vi "atMonochromator_getEvent_SettingsAppliedMonochromatorRanges.vi"(8 "error in (no error)":errorcluster, 11 "logevent_SettingsAppliedMonochromatorRanges_Ctl":T1) -> (0 "error out":errorcluster, 2 "function return":i32, 3 "logevent_SettingsAppliedMonochromatorRanges_Ctl out":T1)   [LabVIEW 2016, in "SALLV_atMonochromator.lvlib"]
doc: "int atMonochromator_shm_getEvent_SettingsAppliedMonochromatorRangesLV(atMonochromator_logevent_SettingsAppliedMonochromatorRangesLV *logevent_SettingsAppliedMonochromatorRanges_Ctl );"
uses:
  SALLV_atMonochromator.lvlib
  DataTypes/logevent_SettingsAppliedMonochromatorRanges.ctl
  SALLV_atMonochromator.so
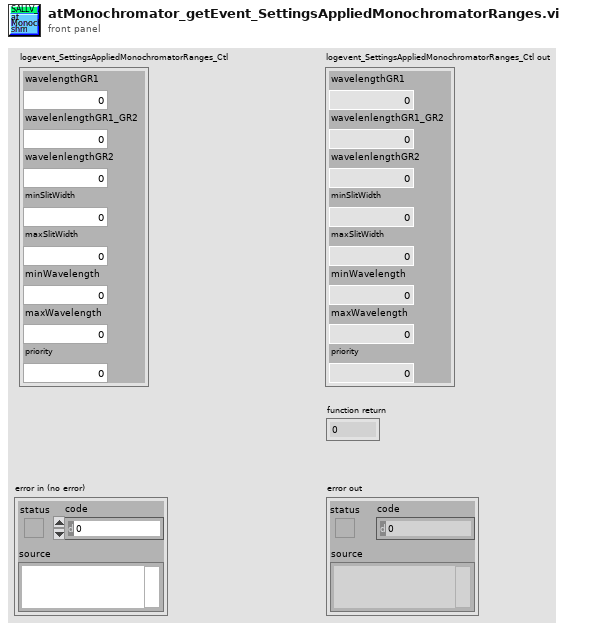
[diagram p1: front panel]
types:
  T1 = typedef "SALLV_atMonochromator.lvlib/logevent_SettingsAppliedMonochromatorRanges.ctl" = cluster{"wavelengthGR1":sgl, "wavelenlengthGR1_GR2":sgl, "wavelenlengthGR2":sgl, "minSlitWidth":sgl, "maxSlitWidth":sgl, "minWavelength":sgl, "maxWavelength":sgl, "priority":i32}
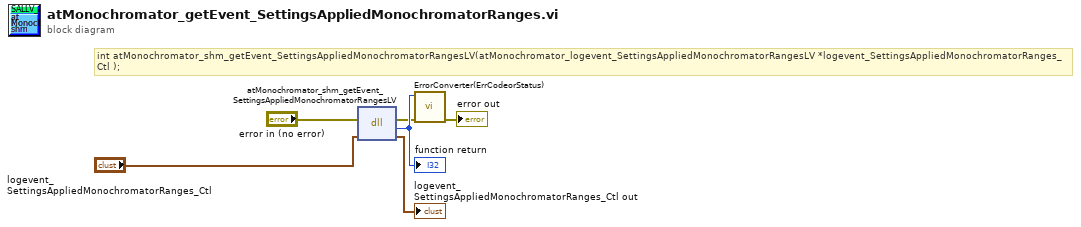
[diagram p0: block diagram]
diagram:
  # "int atMonochromator_shm_getEvent_SettingsAppliedMonochromatorRangesLV(atMonochromator_logevent_SettingsAppliedMonochromatorRangesLV *logevent_SettingsAppliedMonochromatorRanges_Ctl );"
  n1 = dll-call lib="home/andres/Desktop/SAL_atMonochromator/SALLV_atMonochromator.*" fn="atMonochromator_shm_getEvent_SettingsAppliedMonochromatorRangesLV"(error in="error in (no error)", "logevent_SettingsAppliedMonochromatorRanges_Ctl"="logevent_SettingsAppliedMonochromatorRanges_Ctl") -> (error out=w2:errorcluster, w6:i32, "logevent_SettingsAppliedMonochromatorRanges_Ctl"=→"logevent_SettingsAppliedMonochromatorRanges_Ctl out":T1)  [unwired: 2 in, 1 out]
  "function return" <- w6
  n2 = call "ErrorConverter(ErrCodeorStatus).vi"("error in (no error)"=w2, "error code"=w6) -> ("error out"=→"error out":errorcluster)  [unwired: 9 in]
